vi "test Counter Data Plugin Initialize Valid Object.vi"(8 "error in (no error)":errorcluster, 11 "TestCase in":refnum<class "Data Engine Unit Tests.lvclass">) -> (0 "error out":errorcluster, 3 "TestCase out":refnum<class "Data Engine Unit Tests.lvclass">)   [LabVIEW 2017, in "Data Engine Unit Tests.lvclass"]
uses:
  Data Engine Unit Tests.lvclass
  Source/Counter Data Plugin/Counter Data Plugin.lvclass
  D:/xtra/vi/Data Engine/Data Plugin/Data Plugin.lvclass
  <vilib>/addons/_JKI Toolkits/VI Tester/TestCase.llb/TestCase.lvclass
  C:/Program Files/National Instruments/LabVIEW 2017/vi.lib/addons/_JKI Toolkits/VI Tester/TestCase.llb/TestCase.lvclass
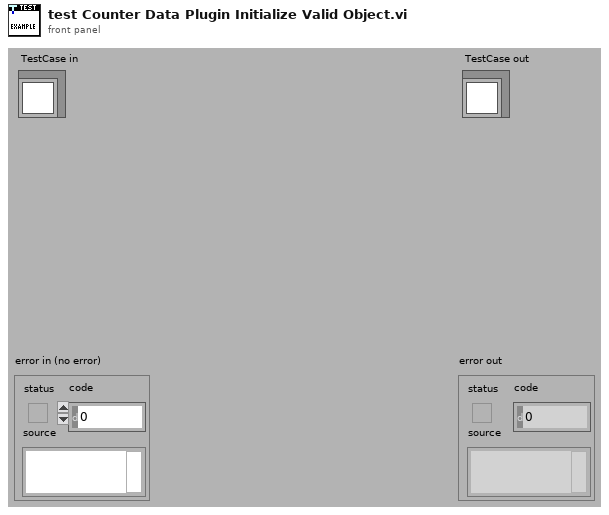
[diagram p1: front panel]
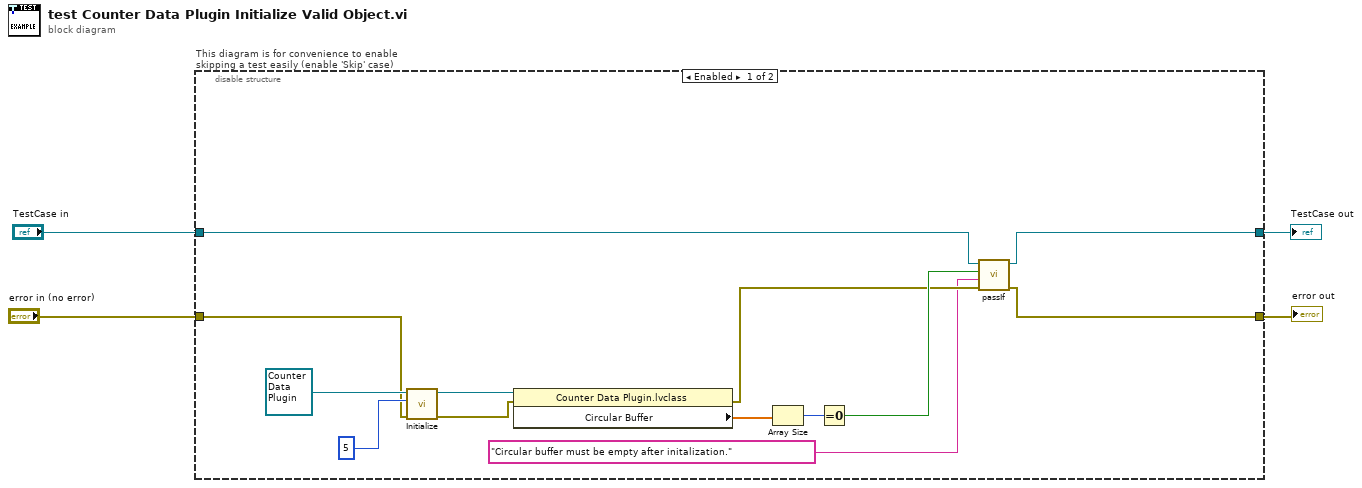
[diagram p0: block diagram]
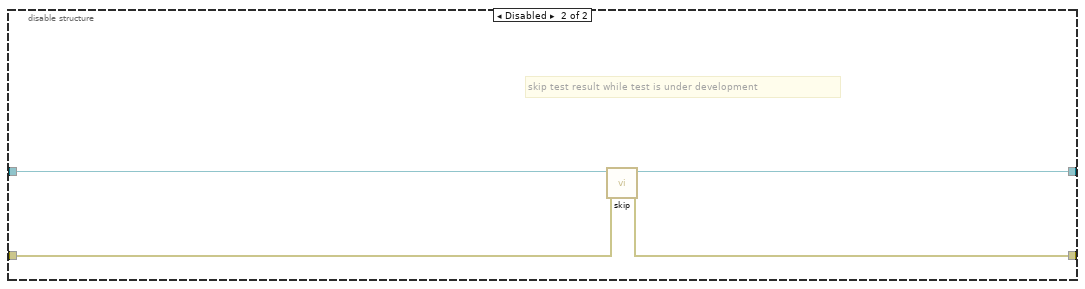
[diagram p2: hidden frame]
diagram:
  n1 = disable-structure "This diagram is for convenience to enable skipping a test easily (enable 'Skip' case)" shown="Enabled" {
    disable-tunnel: "TestCase in" -> [w17 w21]
    disable-tunnel: [w16 w19] -> w1
    disable-tunnel: [w15 w20] -> w3
    disable-tunnel: "error in (no error)" -> [w7 w18]
    frame Enabled {
      n2 = call-dynamic "Initialize.vi"("error in (no error)"=w7, "Circular Buffer Size"=5, "Data Plugin in"=refnum<class "Counter Data Plugin.lvclass"> refnum ("Data Engine.lvlib:Counter Data Plugin.lvclass")) -> ("error out"=w11:errorcluster, "Data Plugin out"=w12:refnum<class "Counter Data Plugin.lvclass">)  [unwired: 7 in]
      n3 = property class="Counter Data Plugin.lvclass"(reference=w12, error in=w11) -> (error out=w6:errorcluster, "Circular Buffer"=w10:dbl[])  [unwired: 1 out]
      n4 = Array Size(array=w10) -> (size(s)=w9:i32)
      n5 = Equal To 0?(x=w9) -> (x = 0?=w8:bool)
      n6 = call-dynamic "passIf.vi"("error in (no error)"=w6, "message (\"\")"="Circular buffer must be empty after initalization." ("message (\"\")"), "pass"=w8, "TestCase in"=w17) -> ("error out"=w15:errorcluster, "TestCase out"=w16:refnum<class "Data Engine Unit Tests.lvclass">)  [unwired: 6 in]
    }
    frame Disabled {
      # "skip test result while test is under development"
      n7 = call <vilib>:"skip.vi"("error in (no error)"=w18, "TestCase in"=w21) -> ("error out"=w20:errorcluster, "TestCase out"=w19:refnum<class "Data Engine Unit Tests.lvclass">)  [unwired: 8 in]
    }
  }
  "error out" <- w3
  "TestCase out" <- w1
